vi "Update Covariance.vi"(8 "R":T1, 9 "H":T1, 10 "K":T1, 11 "Old Covariance":T1) -> (3 "Updated Covariance":T1)   [LabVIEW 2020]
uses:
  <vilib>/Analysis/Matrix/Datatypes/RealMatrix.ctl
  <vilib>/Analysis/7linalg.llb/Real Transpose Matrix.vi
  <vilib>/Analysis/baseanly.llb/Real A x B.vi
  <vilib>/Analysis/7linalg.llb/Create Special Real Matrix.vi
  <vilib>/Analysis/Matrix/Numeric/Subtract/Subtract - RM,RM.vi
  <vilib>/Analysis/Matrix/Numeric/Add/Add - RM,RM.vi
  <vilib>/Analysis/NI_AALPro.lvlib
  <vilib>/Analysis/NI_AALBase.lvlib
  <vilib>/Analysis/Matrix/NI_Matrix.lvlib
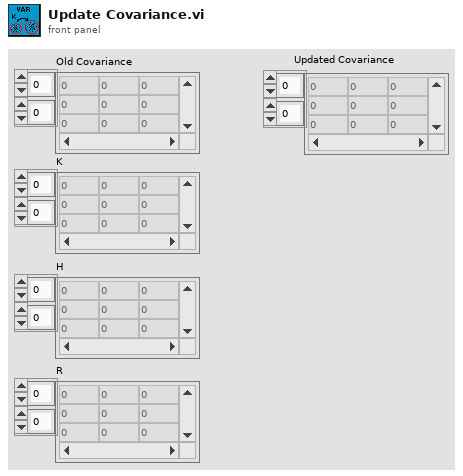
[diagram p1: front panel]
types:
  T1 = typedef "NI_Matrix.lvlib/RealMatrix.ctl" = dbl[][]
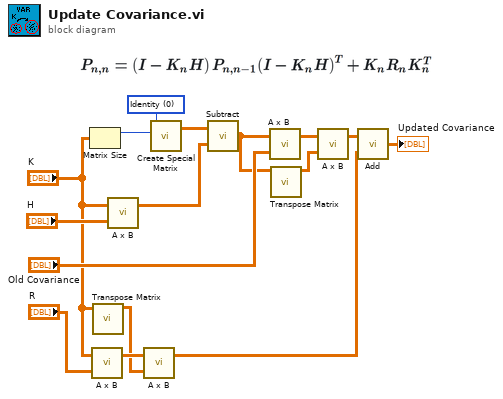
[diagram p0: block diagram]
diagram:
  w16 = 0 items=["Identity", "Diagonal", "Toeplitz", "Vandermonde", "Companion", "Hankel", "Hadamard", "Wilkinson", "Hilbert", "Inverse Hilbert", "Rosser", "Pascal"] ("matrix type")
  n1 = Matrix Size(0:"K") -> (1:w15:i32)  [unwired: 1 out]
  n2 = call-poly <vilib>:"A x B.vi"("B"="R", "A"="K") -> ("A x B"=w5:T1)  [unwired: 1 out]
  n3 = call-poly <vilib>:"Transpose Matrix.vi"("Input Matrix"="K") -> ("Matrix Transpose"=w4:T1)  [unwired: 9 in, 1 out]
  n4 = call-poly <vilib>:"A x B.vi"("B"="H", "A"="K") -> ("A x B"=w12:T1)  [unwired: 1 out]
  n5 = call-poly <vilib>:"A x B.vi"("B"=w4, "A"=w5) -> ("A x B"=w2:T1)  [unwired: 1 out]
  n6 = call-poly <vilib>:"Create Special Matrix.vi"("matrix type"=w16, "matrix size"=w15) -> ("Special Matrix"=w13:T1)  [unwired: 3 in, 1 out]
  n7 = call-poly <vilib>:"Subtract.vi"("Real Matrix B"=w12, "Real Matrix A"=w13) -> ("A - B"=w9:T1)
  n8 = call-poly <vilib>:"A x B.vi"("B"="Old Covariance", "A"=w9) -> ("A x B"=w10:T1)  [unwired: 1 out]
  n9 = call-poly <vilib>:"Transpose Matrix.vi"("Input Matrix"=w9) -> ("Matrix Transpose"=w8:T1)  [unwired: 9 in, 1 out]
  n10 = call-poly <vilib>:"A x B.vi"("B"=w8, "A"=w10) -> ("A x B"=w3:T1)  [unwired: 1 out]
  n11 = call-poly <vilib>:"Add.vi"("Real Matrix B"=w2, "Real Matrix A"=w3) -> ("A + B"=→"Updated Covariance":T1)
